vi "TemperatureControl.vi"() -> ()   [LabVIEW 2011]
uses:
  <vilib>/LabVIEW Interface for Arduino/Type Defs/Arduino Resource.ctl
  <vilib>/LabVIEW Interface for Arduino/Type Defs/Board Type.ctl
  <vilib>/Utility/file.llb/Write To Spreadsheet File (DBL).vi
  <vilib>/express/express arith-compare/Formula/XNode/ExpressFormulaBlockNode.xnode
  <vilib>/LabVIEW Interface for Arduino/LabVIEW Interface for Arduino.lvlib
  <vilib>/addons/control/pid/NI_PID_autopid.lvlib
panel:
  out "Read errors":i32
  out "Temperature (flowcell)":dbl
  in  "file path (dialog if empty)":path=path "L:/BN/ND/Shared/Jordi/Temperature/temp.txt"
  in  "stop":bool
  in  "Equal":bool
  in  "Autotune obj":bool
  in  "Autotune stage":bool
  in  "PID Enabled":bool=TRUE
  in  "instrument handle out":refnum<k15>
  in  "Arduino Resource":T1={"VISA resource"="", "Board Type"=enum."Uno", "Connection Type"=enum."USB / Serial", "Bytes Per Packet (15)"=15}
  out "Stop App":bool
  in  "objective PID gains":T3={"proportional gain (Kc)"=8.0, "integral time (Ti, min)"=2.0, "derivative time (Td, min)"=0.0}
  in  "stage PID gains":T3={"proportional gain (Kc)"=8.0, "integral time (Ti, min)"=2.0, "derivative time (Td, min)"=0.0}
  in  "AutoTunePID":bool caption="Hello"
  in  "Wanted Temp Objective":dbl
  out "Voltage (PSU output) 2":dbl caption="Voltage (output objective)"
  in  "PID output 2":dbl caption="PID Output objective"
  out "Temperature (Arduino input) 2":dbl caption="Temperature (input objective)"
  in  "PID output":dbl caption="PID Output stage"
  out "PSU Output":cluster{"measurement":dbl, "measurement":dbl}(graph)
  out "Arduino input":cluster{sgl, sgl, sgl}(graph)
  out "Temperature (Arduino input)":dbl caption="Temperature (input stage)"
  out "Voltage (PSU output)":dbl caption="Voltage (output stage)"
  in  "Wanted Temp Stage":dbl=35.0
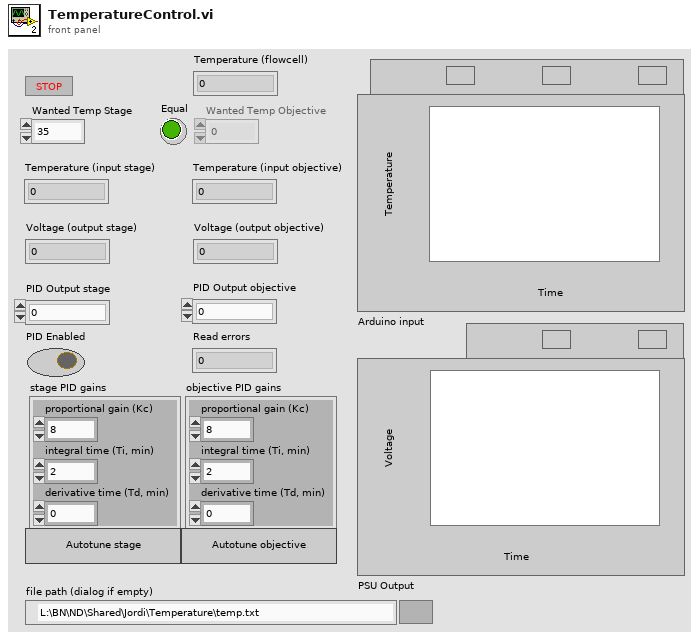
[diagram p1: front panel]
types:
  T1 = typedef "LabVIEW Interface for Arduino.lvlib/Arduino Resource.ctl" = cluster{"VISA resource":refnum<visa-resource-name>, "Board Type":T2, "Connection Type":enum8{"USB / Serial"}, "Bytes Per Packet (15)":u8}
  T2 = typedef "LabVIEW Interface for Arduino.lvlib/Board Type.ctl" = enum16{"Uno", "Dimuelanove w/Atmega 328", "Mega 2560"}
  T3 = cluster{"proportional gain (Kc)":dbl, "integral time (Ti, min)":dbl, "derivative time (Td, min)":dbl}
  T4 = enum8{"Enabled", "Disabled", "Disabled and Grayed Out"}
  T5 = cluster{"proportional gain (Kc)":dbl, "integral time (Ti, min)":dbl, "derivative time (Td, min)":dbl}[]
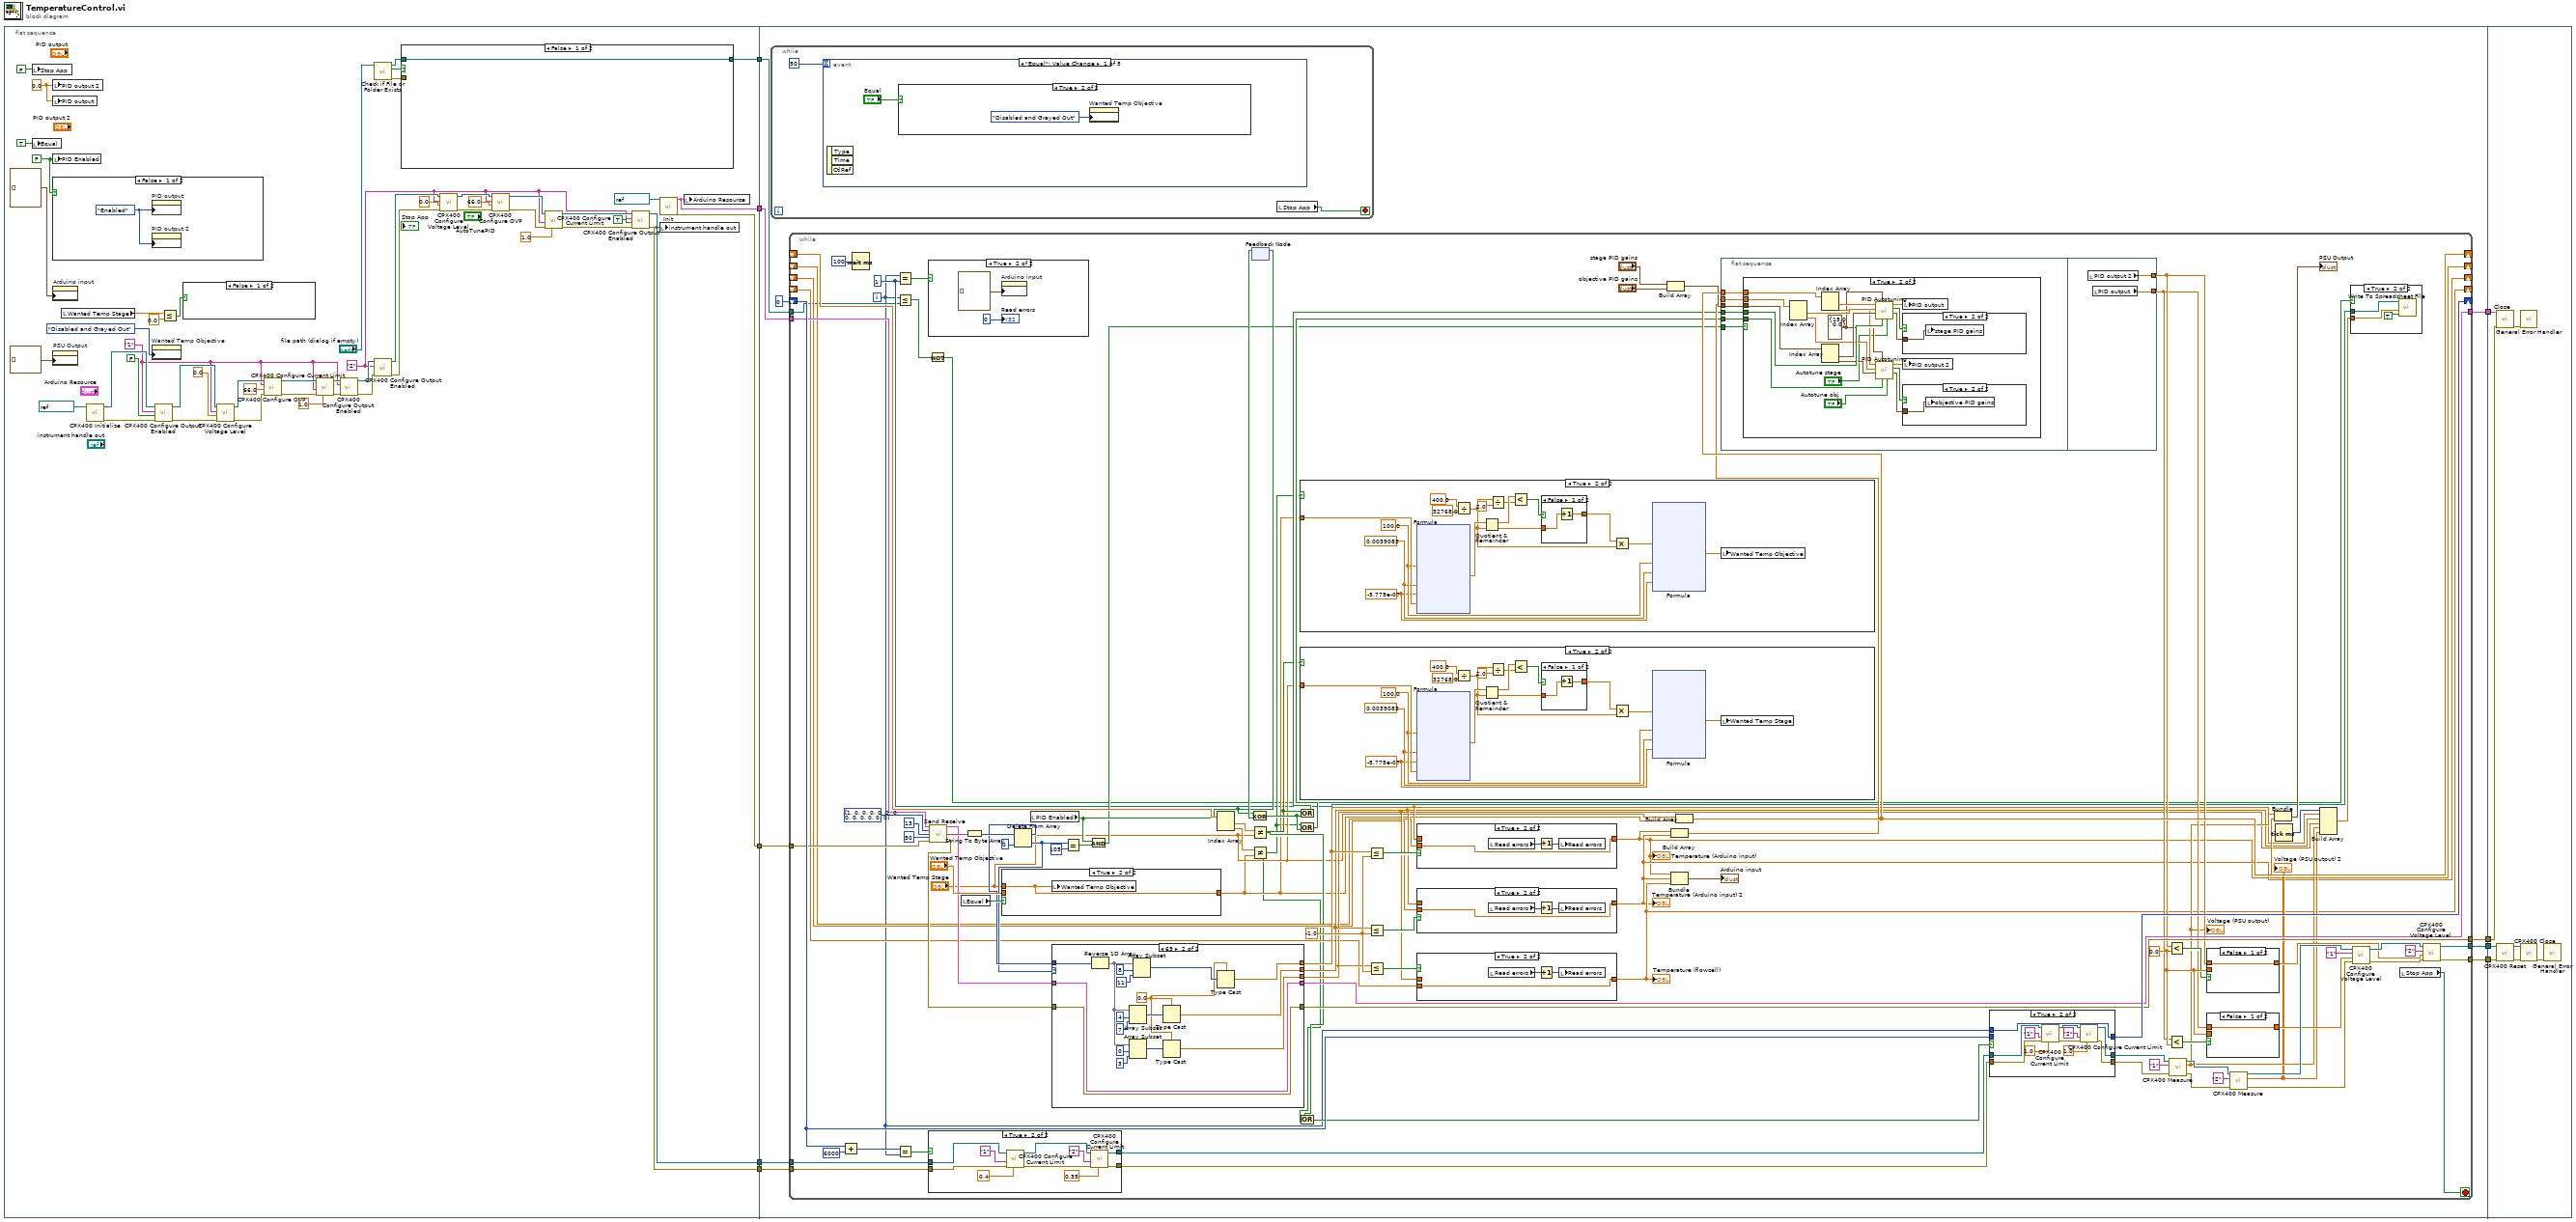
[diagram p0: block diagram]
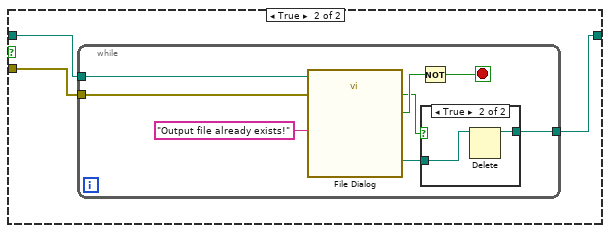
[diagram p2: hidden frame]
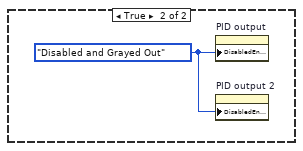
[diagram p4: hidden frame]
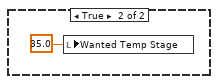
[diagram p5: hidden frame]
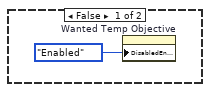
[diagram p6: hidden frame]
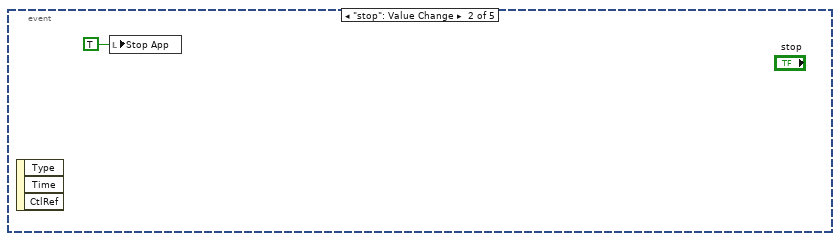
[diagram p7: hidden frame]
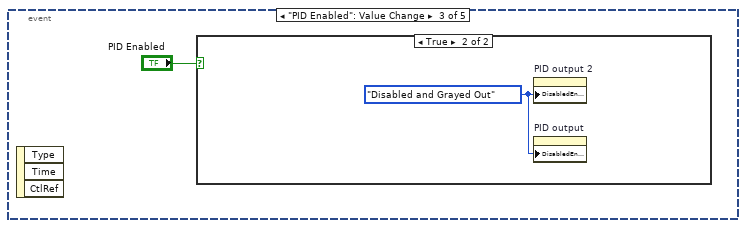
[diagram p8: hidden frame]
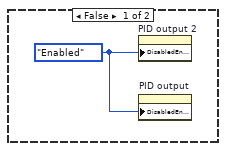
[diagram p9: hidden frame]
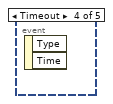
[diagram p10: hidden frame]
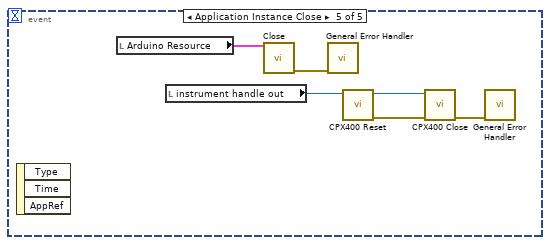
[diagram p11: hidden frame]
diagram:
  n1 = flat-sequence {
    tunnel: [w25] -> w9
    tunnel: [w26] -> w8
    tunnel: [w45] -> w7
    tunnel: [w29] -> w4
    tunnel: [w13] -> w1
    tunnel: w9 -> [w87]
    tunnel: w8 -> [w86]
    tunnel: w7 -> [w85]
    tunnel: [w84] -> w6
    tunnel: [w83] -> w5
    tunnel: w4 -> [w88]
    tunnel: [w81] -> w3
    tunnel: [w80] -> w2
    tunnel: w1 -> [w79]
    tunnel: w6 -> [w398]
    tunnel: w5 -> [w397]
    tunnel: w3 -> [w394]
    tunnel: w2 -> [w393]
    frame #0 {
      w17 = 0.0 ("PID output")
      w18 = FALSE ("PID Enabled")
      w27 = "2" ("channel name (\"1\")")
      w28 = "1" ("channel name (\"1\")")
      n2 = local write "Stop App"(FALSE ("Stop App")) -> ()
      n3 = local write "Equal"(TRUE ("Equal")) -> ()
      n4 = local write "PID output 2"(w17) -> ()
      n5 = local write "PID output"(w17) -> ()
      n6 = local write "PID Enabled"(w18) -> ()
      n7 = case shown="False" w18 {
        frame False {
          w76 = T4."Enabled" ("Disabled")
          n8 = property on="PID output" class="DigNum (strict)"("DisabledEnum"=w76) -> ()  [unwired: 2 in, 2 out]
          n9 = property on="PID output 2" class="DigNum (strict)"("DisabledEnum"=w76) -> ()  [unwired: 2 in, 2 out]
        }
        frame True {
          w77 = T4."Disabled and Grayed Out" ("Disabled")
          n10 = property on="PID output" class="DigNum (strict)"("DisabledEnum"=w77) -> ()  [unwired: 2 in, 2 out]
          n11 = property on="PID output 2" class="DigNum (strict)"("DisabledEnum"=w77) -> ()  [unwired: 2 in, 2 out]
        }
      }
      n12 = property on="Arduino input" class="WFChart (strict)"("History Data"=cluster{sgl, sgl, sgl}[] []) -> ()  [unwired: 2 in, 2 out]
      n13 = property on="PSU Output" class="WFChart (strict)"("History Data"=cluster{"measurement":dbl, "measurement":dbl}[] []) -> ()  [unwired: 2 in, 2 out]
      n14 = local read "Wanted Temp Stage"() -> (w24:dbl)
      n15 = call <instrlib>:"CPX400 Initialize.vi"("resource name"=refnum<k15> "COM4") -> ("error out"=w57:errorcluster, "instrument handle out"=w58:refnum<k15>)  [unwired: 9 in]
      n16 = property on="Wanted Temp Objective" class="DigNum (strict)"("DisabledEnum"=T4."Disabled and Grayed Out" ("Disabled")) -> ()  [unwired: 2 in, 2 out]
      n17 = call <instrlib>:"CPX400 Configure Output Enabled.vi"("error in (no error)"=w57, "enabled (True)"=FALSE, "channel name (\"1\")"=w28, "instrument handle"=w58) -> ("error out"=w55:errorcluster, "instrument handle out"=w56:refnum<k15>)  [unwired: 6 in]
      n18 = Less Or Equal?(x=w24, y=0.0) -> (x <= y?=w22:bool)
      n19 = case shown="False" w22 {
        frame False {
        }
        frame True {
          n20 = local write "Wanted Temp Stage"(35.0 ("Wanted Voltage Stage")) -> ()
        }
      }
      n21 = call <instrlib>:"CPX400 Configure Voltage Level.vi"("error in (no error)"=w55, "level (1.0)"=0.0, "channel name (\"1\")"=w28, "instrument handle"=w56) -> ("error out"=w53:errorcluster, "instrument handle out"=w54:refnum<k15>)  [unwired: 6 in]
      n22 = call <instrlib>:"CPX400 Configure OVP.vi"("error in (no error)"=w53, "limit (66.0)"=66.0, "channel name (\"1\")"=w28, "instrument handle"=w54) -> ("error out"=w51:errorcluster, "instrument handle out"=w52:refnum<k15>)  [unwired: 6 in]
      n23 = call <instrlib>:"CPX400 Configure Current Limit.vi"("limit (1.0)"=1.0, "error in (no error)"=w51, "channel name (\"1\")"=w28, "instrument handle"=w52) -> ("error out"=w49:errorcluster, "instrument handle out"=w50:refnum<k15>)  [unwired: 6 in]
      n24 = call <instrlib>:"CPX400 Configure Output Enabled.vi"("error in (no error)"=w49, "channel name (\"1\")"=w28, "instrument handle"=w50) -> ("error out"=w30:errorcluster, "instrument handle out"=w31:refnum<k15>)  [unwired: 7 in]
      n25 = call <vilib>:"Check if File or Folder Exists.vi"("path"="file path (dialog if empty)") -> ("error out"=w12:errorcluster, "file or folder exists?"=w16:bool, "dup path"=w15:path)  [unwired: 8 in]
      n26 = call <instrlib>:"CPX400 Configure Output Enabled.vi"("error in (no error)"=w30, "channel name (\"1\")"=w27, "instrument handle"=w31) -> ("error out"=w42:errorcluster, "instrument handle out"=w43:refnum<k15>)  [unwired: 7 in]
      n27 = case shown="False" w16 {
        tunnel: w15 -> [w61 w63]
        tunnel: [w61 w64] -> w13
        tunnel: w12 -> [_ w62]
        frame False {
        }
        frame True {
          n28 = while {
            tunnel: [w65] -> w64
            tunnel: w63 -> [w72]
            tunnel: w62 -> [w71]
            stop <- w69 stop-if-true
            n29 = call "File Dialog"("start path"=w72, "prompt"="Output file already exists!", "error in"=w71) -> ("selected path"=w66:path, "exists"=w67:bool, "cancelled"=w70:bool)  [unwired: 9 in, 1 out]
            n30 = Not(x=w70) -> (.not. x?=w69:bool)
            n31 = case shown="True" w67 {
              tunnel: w66 -> [w73 w75]
              tunnel: [w73 w74] -> w65
              frame False {
              }
              frame True {
                n32 = Delete(path (use dialog)=w75) -> (deleted path=w74:path)  [unwired: 4 in, 2 out]
              }
            }
          }
        }
      }
      n33 = call <instrlib>:"CPX400 Configure Voltage Level.vi"("error in (no error)"=w42, "level (1.0)"=0.0, "channel name (\"1\")"=w27, "instrument handle"=w43) -> ("error out"=w40:errorcluster, "instrument handle out"=w41:refnum<k15>)  [unwired: 6 in]
      n34 = call <instrlib>:"CPX400 Configure OVP.vi"("error in (no error)"=w40, "limit (66.0)"=66.0, "channel name (\"1\")"=w27, "instrument handle"=w41) -> ("error out"=w38:errorcluster, "instrument handle out"=w39:refnum<k15>)  [unwired: 6 in]
      n35 = call <instrlib>:"CPX400 Configure Current Limit.vi"("limit (1.0)"=1.0, "error in (no error)"=w38, "channel name (\"1\")"=w27, "instrument handle"=w39) -> ("error out"=w36:errorcluster, "instrument handle out"=w37:refnum<k15>)  [unwired: 6 in]
      n36 = call <instrlib>:"CPX400 Configure Output Enabled.vi"("error in (no error)"=w36, "enabled (True)"=TRUE, "channel name (\"1\")"=w27, "instrument handle"=w37) -> ("error out"=w29:errorcluster, "instrument handle out"=w25:refnum<k15>)  [unwired: 6 in]
      n37 = call <vilib>:"Init.vi"("VISA resource"=refnum<visa-resource-name> "COM3") -> ("Arduino Resource"=w26:T1, "error out"=w45:errorcluster)  [unwired: 17 in]
      n38 = local write "instrument handle out"(w25) -> ()
      n39 = local write "Arduino Resource"(w26) -> ()
    }
    frame #1 {
      n40 = while {
        stop <- w90 stop-if-true
        n41 = event shown="[0] \"Equal\": Value Change" {
          selector: _ -> [_ _ _ _ _]
          dyn-events: _ -> [_ _ _ _ _]
          timeout: 50 -> [_ _ _ _ _]
          event "Equal": Value Change {
            n42 = event-data() -> ()  [unwired: 1 in, 3 out]
            n43 = case shown="True" "Equal" {
              frame False {
                n44 = property on="Wanted Temp Objective" class="DigNum (strict)"("DisabledEnum"=T4."Enabled" ("Disabled")) -> ()  [unwired: 2 in, 2 out]
              }
              frame True {
                n45 = property on="Wanted Temp Objective" class="DigNum (strict)"("DisabledEnum"=T4."Disabled and Grayed Out" ("Disabled")) -> ()  [unwired: 2 in, 2 out]
              }
            }
          }
          event "stop": Value Change {
            n46 = event-data() -> ()  [unwired: 1 in, 3 out]
            n47 = local write "Stop App"(TRUE ("Stop App")) -> ()
          }
          event "PID Enabled": Value Change {
            n48 = event-data() -> ()  [unwired: 1 in, 3 out]
            n49 = case shown="True" "PID Enabled" {
              frame False {
                w96 = T4."Enabled" ("Disabled")
                n50 = property on="PID output 2" class="DigNum (strict)"("DisabledEnum"=w96) -> ()  [unwired: 2 in, 2 out]
                n51 = property on="PID output" class="DigNum (strict)"("DisabledEnum"=w96) -> ()  [unwired: 2 in, 2 out]
              }
              frame True {
                w97 = T4."Disabled and Grayed Out" ("Disabled")
                n52 = property on="PID output 2" class="DigNum (strict)"("DisabledEnum"=w97) -> ()  [unwired: 2 in, 2 out]
                n53 = property on="PID output" class="DigNum (strict)"("DisabledEnum"=w97) -> ()  [unwired: 2 in, 2 out]
              }
            }
          }
          event Timeout {
            n54 = event-data() -> ()  [unwired: 1 in, 2 out]
          }
          event Application Instance Close {
            n55 = event-data() -> ()  [unwired: 1 in, 3 out]
            n56 = local read "Arduino Resource"() -> (w102:T1)
            n57 = local read "instrument handle out"() -> (w98:refnum<k15>)
            n58 = call <vilib>:"Close.vi"("Arduino Resource"=w102) -> ("error out"=w103:errorcluster)  [unwired: 14 in]
            n59 = call <vilib>:"General Error Handler.vi"("error in (no error)"=w103) -> ()  [unwired: 1 in, 14 out]
            n60 = call <instrlib>:"CPX400 Reset.vi"("instrument handle"=w98) -> ("error out"=w99:errorcluster, "instrument handle out"=w100:refnum<k15>)  [unwired: 9 in]
            n61 = call <instrlib>:"CPX400 Close.vi"("error in (no error)"=w99, "instrument handle"=w100) -> ("error out"=w101:errorcluster)  [unwired: 9 in]
            n62 = call <vilib>:"General Error Handler.vi"("error in (no error)"=w101) -> ()  [unwired: 1 in, 14 out]
          }
        }
        n63 = local read "Stop App"() -> (w90:bool)
      }
      n64 = while {
        tunnel: w88 -> [w195]
        tunnel: w87 -> [w196]
        tunnel: w86 -> [w144]
        tunnel: w85 -> [w143]
        tunnel: [w142] -> w84
        tunnel: [w141] -> w83
        shift-right: [w194] -> _
        shift-left: 0 -> [w193]
        tunnel: [w180] -> w81
        tunnel: [w179] -> w80
        shift-right: [w178] -> _
        shift-left: _ -> [w177]
        shift-right: [w120] -> _
        shift-left: _ -> [w119]
        shift-right: [w118] -> _
        shift-left: _ -> [w117]
        shift-right: [w116] -> _
        shift-left: _ -> [w115]
        tunnel: w79 -> [w110]
        i -> [w107]
        stop <- w104 stop-if-true
        w124 = -1.0 ("y")
        w108 = 1 ("y")
        w173 = 0.0 ("y")
        n65 = Add(x=w193, y=6000) -> (x+y=w168:i32)
        n66 = Wait (ms)(milliseconds to wait=u32 100) -> ()  [unwired: 1 out]
        n67 = Equal?(x=w107, y=w108) -> (x = y?=w140:bool)
        n68 = Less Or Equal?(x=w107, y=w108) -> (x <= y?=w106:bool)
        n69 = Equal?(x=w168, y=w107) -> (x = y?=w167:bool)
        n70 = case shown="True" w140 {
          frame False {
          }
          frame True {
            n71 = property on="Arduino input" class="WFChart (strict)"("History Data"=cluster{sgl, sgl, sgl}[] []) -> ()  [unwired: 2 in, 2 out]
            "Read errors" <- 0 ("Read errors")
          }
        }
        n72 = case shown="True" w167 {
          tunnel: [w377 w388] -> w171
          tunnel: w196 -> [w377 w382]
          tunnel: w195 -> [w378 w381]
          tunnel: [w378 w387] -> w170
          frame False {
          }
          frame True {
            n73 = call <instrlib>:"CPX400 Configure Current Limit.vi"("limit (1.0)"=0.4, "error in (no error)"=w381, "channel name (\"1\")"="1" ("channel name (\"1\")"), "instrument handle"=w382) -> ("error out"=w383:errorcluster, "instrument handle out"=w384:refnum<k15>)  [unwired: 6 in]
            n74 = call <instrlib>:"CPX400 Configure Current Limit.vi"("limit (1.0)"=0.35, "error in (no error)"=w383, "channel name (\"1\")"="2" ("channel name (\"1\")"), "instrument handle"=w384) -> ("error out"=w387:errorcluster, "instrument handle out"=w388:refnum<k15>)  [unwired: 6 in]
          }
        }
        n75 = Not(x=w106) -> (.not. x?=w105:bool)
        n76 = call <vilib>:"Send Receive.vi"("Arduino Resource"=w144, "Data"=u8[] [1, 0, 0, 0, 0, 0, 0, 0, 0, 0, 0, 0, 0], "Bytes To Read (0)"=u8 13, "Time Out (100 ms)"=50, "error in"=w143) -> ("Arduino Resource"=w145:T1, "Read Buffer"=w150:string, "error out"=w146:errorcluster)  [unwired: 8 in]
        n77 = local read "Equal"() -> (w159:bool)
        n78 = String To Byte Array(string=w150) -> (unsigned byte array=w149:u8[])
        n79 = case shown="True" w159 {
          tunnel: [w361 w362] -> w112
          tunnel: "Wanted Temp Stage" -> [_ w362]
          tunnel: "Wanted Temp Objective" -> [w361 _]
          frame False {
          }
          frame True {
            n80 = local write "Wanted Temp Objective"(w362) -> ()
          }
        }
        n81 = Delete From Array(array=w149, index=0) -> (deleted portion=w134:u8, array with subset deleted=w147:u8[])  [unwired: 1 in]
        n82 = local read "PID Enabled"() -> (w136:bool)
        n83 = case shown="69" w134 {
          tunnel: w147 -> [_ w324]
          tunnel: [w309 w314] -> w123
          tunnel: w146 -> [w312 w330]
          tunnel: [w311 w330] -> w141
          tunnel: w145 -> [w310 w329]
          tunnel: [w310 w329] -> w142
          tunnel: [w309 w315] -> w122
          tunnel: [w309 w316] -> w121
          frame 0, Default {
            w309 = sgl -2.0
            n84 = Unbundle By Name(w310) -> ("VISA resource"=w313:refnum<visa-resource-name>)
            n85 = VISA Flush I/O Buffer(VISA resource name=w313, error in (no error)=w312) -> (error out=w311:errorcluster)  [unwired: 1 in, 1 out]
          }
          frame 105 {
            w318 = sgl 0.0
            n86 = Reverse 1D Array(array=w324) -> (reversed array=w321:u8[])
            n87 = Array Subset(array=w321, index=4, length=7) -> (w323:u8[])
            n88 = Array Subset(array=w321, index=0, length=3) -> (w317:u8[])
            n89 = Array Subset(array=w321, index=8, length=11) -> (w322:u8[])
            n90 = Type Cast(type=w318, x=w323) -> (*(type *) &x=w315:sgl)
            n91 = Type Cast(type=w318, x=w317) -> (*(type *) &x=w316:sgl)
            n92 = Type Cast(type=w318, x=w322) -> (*(type *) &x=w314:sgl)
          }
        }
        n93 = Equal?(x=w134, y=u8 105) -> (x = y?=w132:bool)
        n94 = And(x=w136, y=w132) -> (x .and. y?=w135:bool)
        n95 = Index Array(array=w177) -> (element #1=w162:dbl, element #2=w161:dbl)  [unwired: 2 in]
        n96 = feedback-in #1(w136) -> ()
        n97 = feedback #1() -> (w154:bool)  [unwired: 1 in]
        n98 = Exclusive Or(1:w154, 2:w136) -> (0:w153:bool)
        n99 = Not Equal?(x=w162, y="Wanted Temp Stage") -> (x != y?=w114:bool)
        n100 = Not Equal?(x=w161, y=w112) -> (x != y?=w111:bool)
        n101 = Or(x=w114, y=w153) -> (x .or. y?=w156:bool)
        n102 = Or(x=w111, y=w153) -> (x .or. y?=w155:bool)
        n103 = Or(x=w114, y=w111) -> (x .or. y?=w160:bool)
        n104 = case shown="True" w111 {
          tunnel: w112 -> [_ w216]
          frame False {
          }
          frame True {
            w213 = 100.0 ("y")
            w212 = 0.0039083 ("y")
            w211 = -5.775e-07 ("y")
            n105 = xnode "Formula"("R0"=w213, "A"=w212, "B"=w211, "T"=w216) -> ("Result"=w215:dbl)  [unwired: 1 in, 1 out]
            n106 = Divide(x=400.0, y=32768.0) -> (x/y=w207:dbl)
            n107 = Quotient & Remainder(x=w215, y=w207) -> (x-y*floor(x/y)=w208:dbl, floor(x/y)=w203:dbl)
            n108 = Divide(x=w207, y=2.0) -> (x/y=w205:dbl)
            n109 = Less?(x=w208, y=w205) -> (x < y?=w204:bool)
            n110 = case shown="False" w204 {
              tunnel: w203 -> [w218 w219]
              tunnel: [w217 w219] -> w202
              frame False {
                n111 = Increment(x=w218) -> (x+1=w217:dbl)
              }
              frame True {
              }
            }
            n112 = Multiply(x=w202, y=w207) -> (x*y=w214:dbl)
            n113 = xnode "Formula"("R"=w214, "R0"=w213, "A"=w212, "B"=w211) -> ("Result"=w201:dbl)  [unwired: 1 in, 1 out]
            n114 = local write "Wanted Temp Objective"(w201) -> ()
          }
        }
        n115 = case shown="True" w114 {
          tunnel: "Wanted Temp Stage" -> [_ w263]
          frame False {
          }
          frame True {
            w260 = 100.0 ("y")
            w259 = 0.0039083 ("y")
            w258 = -5.775e-07 ("y")
            n116 = xnode "Formula"("R0"=w260, "A"=w259, "B"=w258, "T"=w263) -> ("Result"=w262:dbl)  [unwired: 1 in, 1 out]
            n117 = Divide(x=400.0, y=32768.0) -> (x/y=w254:dbl)
            n118 = Quotient & Remainder(x=w262, y=w254) -> (x-y*floor(x/y)=w255:dbl, floor(x/y)=w250:dbl)
            n119 = Divide(x=w254, y=2.0) -> (x/y=w252:dbl)
            n120 = Less?(x=w255, y=w252) -> (x < y?=w251:bool)
            n121 = case shown="False" w251 {
              tunnel: w250 -> [w265 w266]
              tunnel: [w264 w266] -> w249
              frame False {
                n122 = Increment(x=w265) -> (x+1=w264:dbl)
              }
              frame True {
              }
            }
            n123 = Multiply(x=w249, y=w254) -> (x*y=w261:dbl)
            n124 = xnode "Formula"("R"=w261, "R0"=w260, "A"=w259, "B"=w258) -> ("Result"=w248:dbl)  [unwired: 1 in, 1 out]
            n125 = local write "Wanted Temp Stage"(w248) -> ()
          }
        }
        n126 = Less Or Equal?(x=w123, y=w124) -> (x <= y?=w127:bool)
        n127 = Less Or Equal?(x=w122, y=w124) -> (x <= y?=w126:bool)
        n128 = Less Or Equal?(x=w121, y=w124) -> (x <= y?=w125:bool)
        n129 = case shown="True" w127 {
          tunnel: w123 -> [w299 _]
          tunnel: [w299 w302] -> w116
          tunnel: w115 -> [_ w302]
          frame False {
          }
          frame True {
            n130 = local read "Read errors"() -> (w301:i32)
            n131 = Increment(x=w301) -> (x+1=w300:i32)
            n132 = local write "Read errors"(w300) -> ()
          }
        }
        "Temperature (Arduino input)" <- w116
        n133 = case shown="True" w126 {
          tunnel: w122 -> [w303 _]
          tunnel: [w303 w306] -> w118
          tunnel: w117 -> [_ w306]
          frame False {
          }
          frame True {
            n134 = local read "Read errors"() -> (w305:i32)
            n135 = Increment(x=w305) -> (x+1=w304:i32)
            n136 = local write "Read errors"(w304) -> ()
          }
        }
        "Temperature (Arduino input) 2" <- w118
        n137 = case shown="True" w125 {
          tunnel: [w295 w298] -> w120
          tunnel: w121 -> [w295 _]
          tunnel: w119 -> [_ w298]
          frame False {
          }
          frame True {
            n138 = local read "Read errors"() -> (w297:i32)
            n139 = Increment(x=w297) -> (x+1=w296:i32)
            n140 = local write "Read errors"(w296) -> ()
          }
        }
        "Temperature (flowcell)" <- w120
        n141 = Build Array("stage PID gains", "objective PID gains") -> (w164:T5)
        n142 = Build Array(w116, w118) -> (w163:sgl[])
        n143 = Bundle(w116, w118, w120) -> (→"Arduino input":cluster{sgl, sgl, sgl})  [unwired: 1 in]
        n144 = Build Array("Wanted Temp Stage", w112) -> (w178:dbl[])
        n145 = flat-sequence {
          tunnel: w178 -> [w336]
          tunnel: w164 -> [w335]
          tunnel: w163 -> [w334]
          tunnel: w135 -> [w333]
          tunnel: w155 -> [w332]
          tunnel: w156 -> [w331]
          tunnel: [w360] -> w137
          tunnel: [w359] -> w138
          frame #0 {
            n146 = case shown="True" w333 {
              tunnel: w335 -> [_ w351]
              tunnel: w336 -> [_ w355]
              tunnel: w334 -> [_ w353]
              tunnel: w331 -> [_ w356]
              tunnel: w332 -> [_ w342]
              frame False {
              }
              frame True {
                w341 = cluster{"output high":dbl, "output low":dbl} {"output high"=15.0, "output low"=0.0} ("output range")
                n147 = Index Array(array=w353) -> (element #1=w352:sgl, element #2=w346:sgl)  [unwired: 2 in]
                n148 = Index Array(array=w355) -> (element #1=w354:dbl, element #2=w347:dbl)  [unwired: 2 in]
                n149 = Index Array(array=w351) -> (element #1=w350:T3, element #2=w345:T3)  [unwired: 2 in]
                n150 = call <vilib>:"PID Autotuning.vi"("autotune? (F)"="Autotune stage", "reinitialize? (F)"=w356, "output range"=w341, "PID gains"=w350, "process variable"=w352, "setpoint"=w354) -> ("PID gains out"=w348:T3, "tuning completed?"=w349:bool, "output"=w337:dbl)  [unwired: 2 in, 1 out]
                n151 = call <vilib>:"PID Autotuning.vi"("autotune? (F)"="Autotune obj", "reinitialize? (F)"=w342, "output range"=w341, "PID gains"=w345, "process variable"=w346, "setpoint"=w347) -> ("PID gains out"=w343:T3, "tuning completed?"=w344:bool, "output"=w338:dbl)  [unwired: 2 in, 1 out]
                n152 = local write "PID output"(w337) -> ()
                n153 = case shown="True" w349 {
                  tunnel: w348 -> [_ w358]
                  frame False {
                  }
                  frame True {
                    n154 = local write "stage PID gains"(w358) -> ()
                  }
                }
                n155 = local write "PID output 2"(w338) -> ()
                n156 = case shown="True" w344 {
                  tunnel: w343 -> [_ w357]
                  frame False {
                  }
                  frame True {
                    n157 = local write "objective PID gains"(w357) -> ()
                  }
                }
              }
            }
          }
          frame #1 {
            n158 = local read "PID output 2"() -> (w359:dbl)
            n159 = local read "PID output"() -> (w360:dbl)
          }
        }
        n160 = case shown="True" w160 {
          tunnel: w171 -> [w365 w369]
          tunnel: w170 -> [w364 w370]
          tunnel: [w364 w366] -> w157
          tunnel: [w365 w376] -> w183
          tunnel: w107 -> [_ w374]
          tunnel: [w363 w374] -> w194
          tunnel: w193 -> [w363 _]
          frame False {
          }
          frame True {
            n161 = call <instrlib>:"CPX400 Configure Current Limit.vi"("limit (1.0)"=1.0, "error in (no error)"=w370, "channel name (\"1\")"="1" ("channel name (\"1\")"), "instrument handle"=w369) -> ("error out"=w371:errorcluster, "instrument handle out"=w372:refnum<k15>)  [unwired: 6 in]
            n162 = call <instrlib>:"CPX400 Configure Current Limit.vi"("limit (1.0)"=1.0, "error in (no error)"=w371, "channel name (\"1\")"="2" ("channel name (\"1\")"), "instrument handle"=w372) -> ("error out"=w366:errorcluster, "instrument handle out"=w376:refnum<k15>)  [unwired: 6 in]
          }
        }
        n163 = Less?(x=w138, y=w173) -> (x < y?=w172:bool)
        n164 = Less?(x=w137, y=w173) -> (x < y?=w176:bool)
        n165 = call <instrlib>:"CPX400 Measure.vi"("error in (no error)"=w157, "channel name (\"1\")"="1" ("channel name (\"1\")"), "instrument handle"=w183) -> ("error out"=w192:errorcluster, "measurement"=w129:dbl, "instrument handle out"=w191:refnum<k15>)  [unwired: 6 in]
        "Voltage (PSU output)" <- w129
        n166 = case shown="False" w172 {
          tunnel: [w389 w390] -> w174
          tunnel: w173 -> [_ w390]
          tunnel: w138 -> [w389 _]
          frame False {
          }
          frame True {
          }
        }
        n167 = case shown="False" w176 {
          tunnel: [w391 w392] -> w175
          tunnel: w173 -> [_ w392]
          tunnel: w137 -> [w391 _]
          frame False {
          }
          frame True {
          }
        }
        n168 = call <instrlib>:"CPX400 Measure.vi"("error in (no error)"=w192, "channel name (\"1\")"="2" ("channel name (\"1\")"), "instrument handle"=w191) -> ("error out"=w181:errorcluster, "measurement"=w128:dbl, "instrument handle out"=w182:refnum<k15>)  [unwired: 6 in]
        "Voltage (PSU output) 2" <- w128
        n169 = Bundle("measurement"=w129, "measurement"=w128) -> (→"PSU Output":cluster{"measurement":dbl, "measurement":dbl})  [unwired: 1 in]
        n170 = Tick Count (ms)() -> (millisecond timer value=w131:u32)
        n171 = Build Array(w131, w123, w122, w121, w129, w128) -> (w109:dbl[])
        n172 = case shown="True" w105 {
          tunnel: w110 -> [_ w200]
          tunnel: w109 -> [_ w199]
          frame False {
          }
          frame True {
            n173 = call-poly <vilib>:"Write To Spreadsheet File.vi"("append to file? (new file:F)"=TRUE, "1D data"=w199, "file path (dialog if empty)"=w200) -> ()  [unwired: 5 in, 1 out]
          }
        }
        n174 = call <instrlib>:"CPX400 Configure Voltage Level.vi"("error in (no error)"=w181, "level (1.0)"=w175, "channel name (\"1\")"="1" ("channel name (\"1\")"), "instrument handle"=w182) -> ("error out"=w187:errorcluster, "instrument handle out"=w188:refnum<k15>)  [unwired: 6 in]
        n175 = local read "Stop App"() -> (w104:bool)
        n176 = call <instrlib>:"CPX400 Configure Voltage Level.vi"("error in (no error)"=w187, "level (1.0)"=w174, "channel name (\"1\")"="2" ("channel name (\"1\")"), "instrument handle"=w188) -> ("error out"=w179:errorcluster, "instrument handle out"=w180:refnum<k15>)  [unwired: 6 in]
      }
    }
    frame #2 {
      n177 = call <vilib>:"Close.vi"("Arduino Resource"=w398, "error in"=w397) -> ("error out"=w399:errorcluster)  [unwired: 13 in]
      n178 = call <instrlib>:"CPX400 Reset.vi"("error in (no error)"=w393, "instrument handle"=w394) -> ("error out"=w395:errorcluster, "instrument handle out"=w396:refnum<k15>)  [unwired: 8 in]
      n179 = call <vilib>:"General Error Handler.vi"("error in (no error)"=w399) -> ()  [unwired: 1 in, 14 out]
      n180 = call <instrlib>:"CPX400 Close.vi"("error in (no error)"=w395, "instrument handle"=w396) -> ("error out"=w400:errorcluster)  [unwired: 9 in]
      n181 = call <vilib>:"General Error Handler.vi"("error in (no error)"=w400) -> ()  [unwired: 1 in, 14 out]
    }
  }
